vi "Query_Dust_Event_v2.vi"(8 "error in (no error)":errorcluster, 9 "Save Waveforms":bool) -> (0 "error out":errorcluster)   [LabVIEW 2013]
uses:
  Private/Constraints.ctl
  Private/Graph.ctl
  <vilib>/Utility/miscctls.llb/LVPointTypeDef.ctl
  <vilib>/Utility/error.llb/DialogType.ctl
  <userlib>/_OpenG.lib/array/array.llb/Remove Duplicates from 1D Array (String)__ogtk.vi
  <userlib>/_OpenG.lib/array/array.llb/Remove Duplicates from 1D Array (DBL)__ogtk.vi
  <vilib>/Utility/file.llb/Write To Spreadsheet File (string).vi
  Private/Global graph.vi
panel:
  out "Open plot windows":refnum<vi>[](array[refnum])
  out "Week":dbl
  out "Last Metadata Name":string
  out "Density":dbl
  out "Names":string[](array[string])
  in  "write metadata only":bool
  in  "Tab Control":T1(tab)
  in  "Limit to":dbl=10000.0
  in  "Limit plotted events":bool
  in  "Reset Scale to Default":bool
  in  "Experiment Group":string
  in  "Plot":bool
  in  "Select Names":bool
  in  "Save Metadata":bool
  in  "Show Names":bool
  out "Metadata Slide":u8(slide) scale=0.0..100.0
  in  "Save Image":bool
  in  "Plot Radius?":bool
  out "Constrained Distribution":T2
  in  "Experiment Name":string
  out "Waveforms Slide":u8(slide) scale=0.0..100.0
  in  "Reset Constraints to Default":bool
  in  "New Plot Window":bool
  out "Number of Matching Events:":i32
  out "Description for Experiment Name:":string caption="Experiment Description:"
  out "Percentage of triggers that fit constraints:":dbl format="%#_4g%"
  out "Total Number of triggers:":i64
  in  "Constraints":T3 {"Estimate Quality" scale=0.0..5.0; "Lower Mass Limit (kg)" min=0.0 step=1e-20; "Upper Mass Limit (kg)" min=0.0 step=1e-20}
  out "Dust Type":string
  in  "Radius (µm)":dbl=1.9999993051655787
  in  "Mass (kg)":dbl=2.6386e-13 min=1e-20 max=1e-10
  in  "Velocity (km/s)":dbl=1.0 min=0.1 max=200.0
  in  "Sensitivity:":dbl=12100000000000.0
  in  "Vnoise Estimate:":dbl=0.005
  in  "Pelletron Voltage (MV):":dbl=2.0
  out "Test":bool caption="Test Database in use:"
  out "Test 2":bool caption="Production Database in use:"
  in  "Exit":bool
  # "Query Dust Event 2.0"
  # "Cursor"
  # "events"
  # "Plot Settings:"
  # "Error Status:"
  # "ODBC Connection Status:"
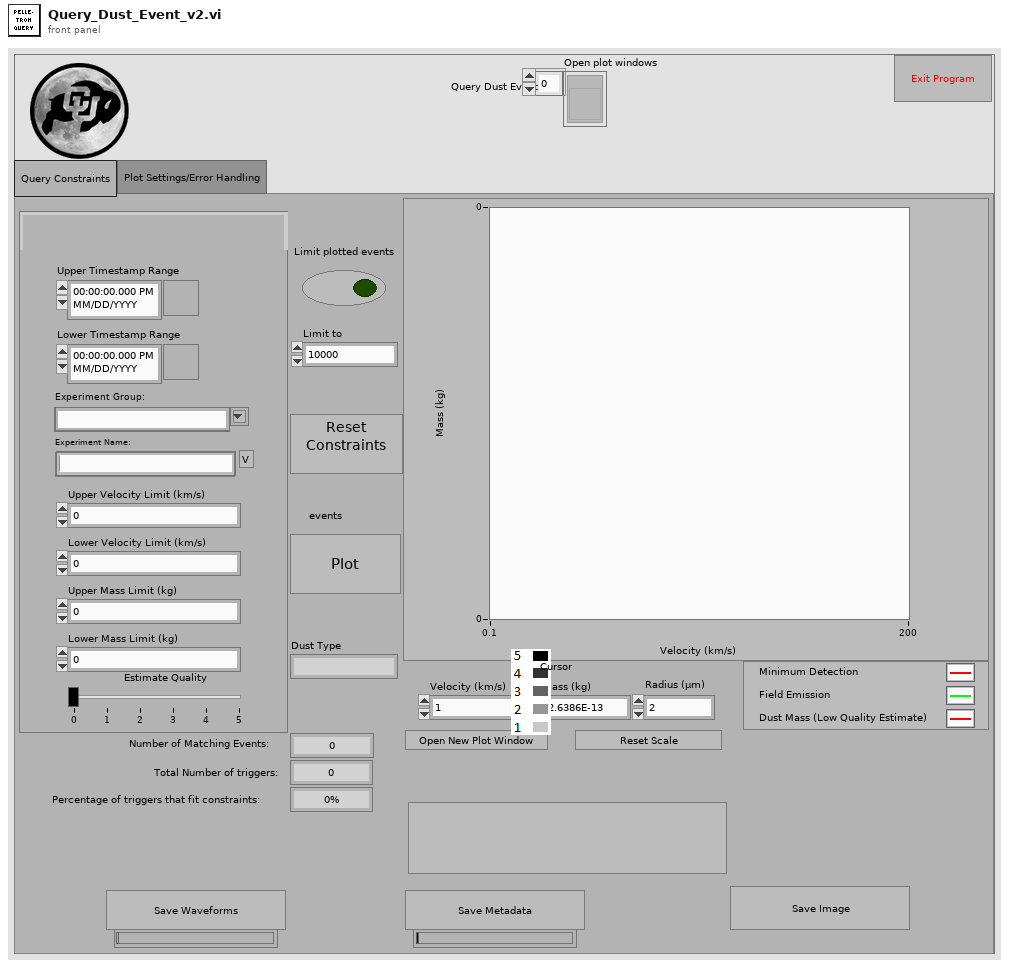
[diagram p1: front panel]
types:
  T1 = enum32{"Query Constraints", "Plot Settings/Error Handling"}
  T2 = typedef "Graph.ctl" = cluster{cluster{"Vnoise":dbl, "Vnoise":dbl}[]}[]
  T3 = typedef "Constraints.ctl" = cluster{"Upper Timestamp Range":timestamp, "Lower Timestamp Range":timestamp, "Experiment Group:":string, "Experiment Name:":i32[], "Upper Velocity Limit (km/s)":dbl, "Lower Velocity Limit (km/s)":dbl, "Upper Mass Limit (kg)":dbl, "Lower Mass Limit (kg)":dbl, "name array":string[], "Estimate Quality":cluster{dbl, dbl}}
  T4 = typedef "LVPointTypeDef.ctl" = cluster{"Horizontal":i16, "Vertical":i16}
  T5 = typedef "Query_Dust_Event.ctl" = cluster{"Dust Event ID":i64, "Integer Timestamp":i64, "Velocity":sgl, "Mass":sgl, "Charge":sgl, "Radius":sgl, "Passed_3rd_Detector":i8, "High Voltage":sgl, "+ High Voltage Supply":sgl, "- High Voltage Supply":sgl, "HV Control Difference":sgl, "Vacuum Pressure":sgl, "Radiation":sgl, "Column Current":sgl, "Lost Charge":sgl, "Chain Current":sgl, "Control High Voltage":sgl, "Current Group ID:":string, "Current Experiment Name:":string, "Current Experiment Description:":string, "Estimate Source":T6, "Estimate Quality":sgl, "File Location":T7, "Dust Type":string, "Dust Density":sgl}
  T6 = typedef "Estimate_source.ctl" = i8
  T7 = typedef "File_location.ctl" = i8
  T8 = enum8{"Enabled", "Disabled", "Disabled and Grayed Out"}
  T9 = enum16{"Left Button", "Center Button", "Right Button", "Window Close"}
  T10 = typedef "NI_Database_API.lvlib/Conn ObjectReference.ctl" = refnum<k1>
  T11 = typedef "DialogType.ctl" = u16
  T12 = typedef "Post_Signal.ctl" = cluster{"Integer Timestamp":i64, "Dust Event ID":i64, "Role ID":T13, "Data":sgl[], "Signal Length":i32, "dt":sgl, "Offset":dbl, "Hardware ID":T14}
  T13 = typedef "Role ID.ctl" = enum16{"First_Detector", "Second_Detector", "Third_Detector", "LeCroy_CH1", "LeCroy_CH2", "LeCroy_CH3", "LeCroy_CH4", "PSU"}
  T14 = typedef "Hardware ID.ctl" = enum16{"Unknown", "CSA 1", "CSA 2", "CSA 3", "CSA 4", "CSA 5", "CSA 6"}
  T15 = typedef "imagedata.ctl" = cluster{"image type":i32, "image depth":i32, "image":u8[], "mask":u8[], "colors":u32[], "Rectangle":cluster{"left":i16, "top":i16, "right":i16, "bottom":i16}}
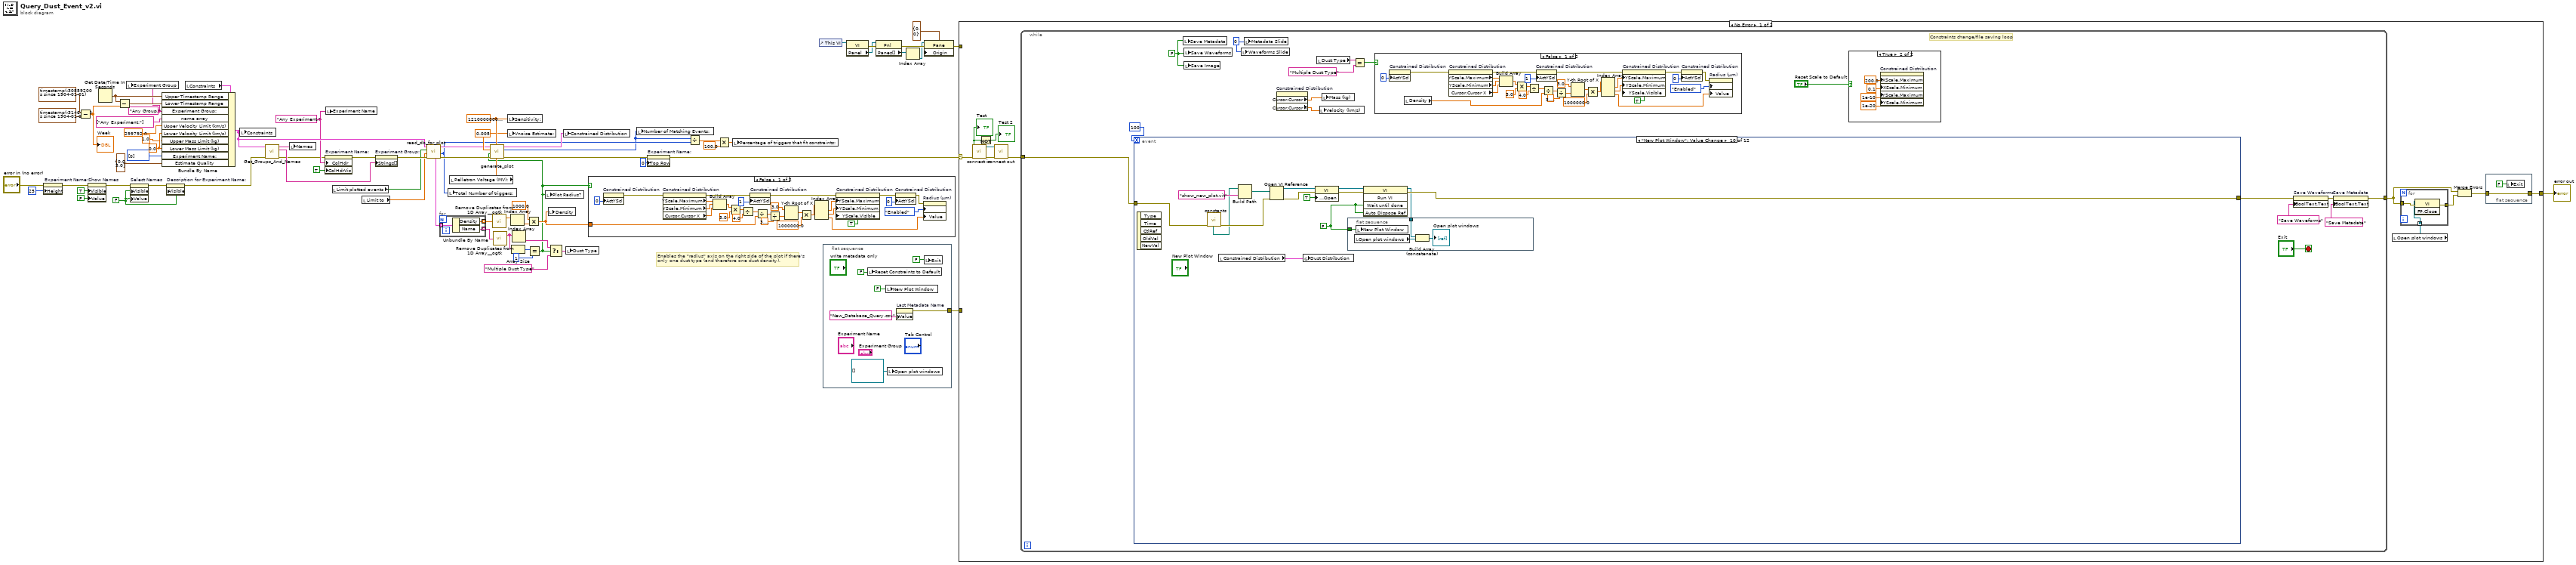
[diagram p0: block diagram]
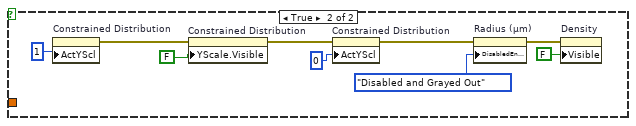
[diagram p2: hidden frame]
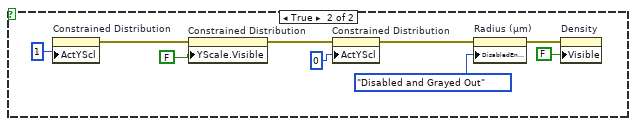
[diagram p3: hidden frame]
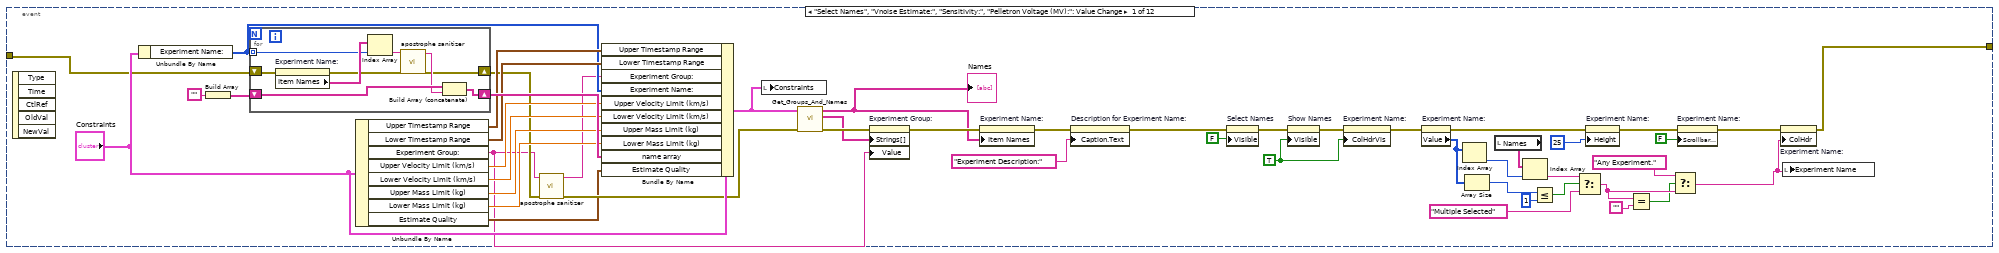
[diagram p5: hidden frame]
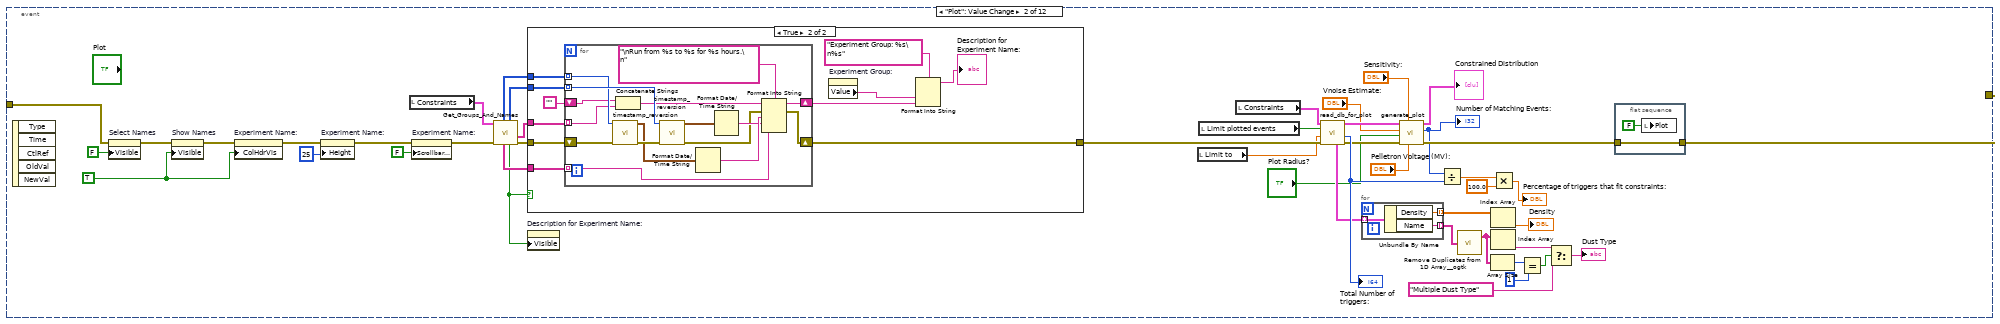
[diagram p6: hidden frame]
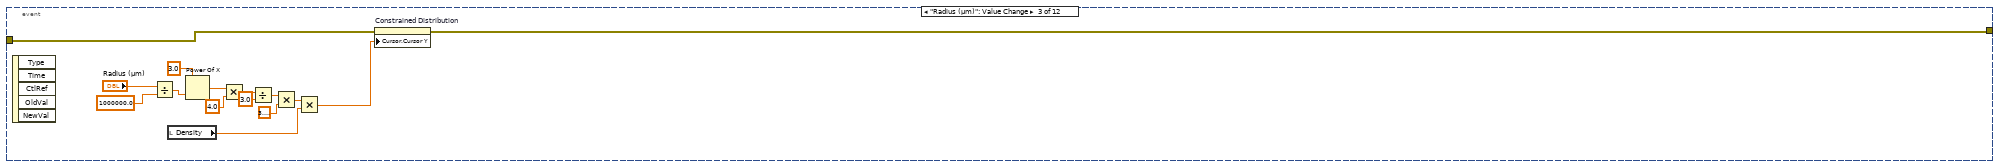
[diagram p8: hidden frame]
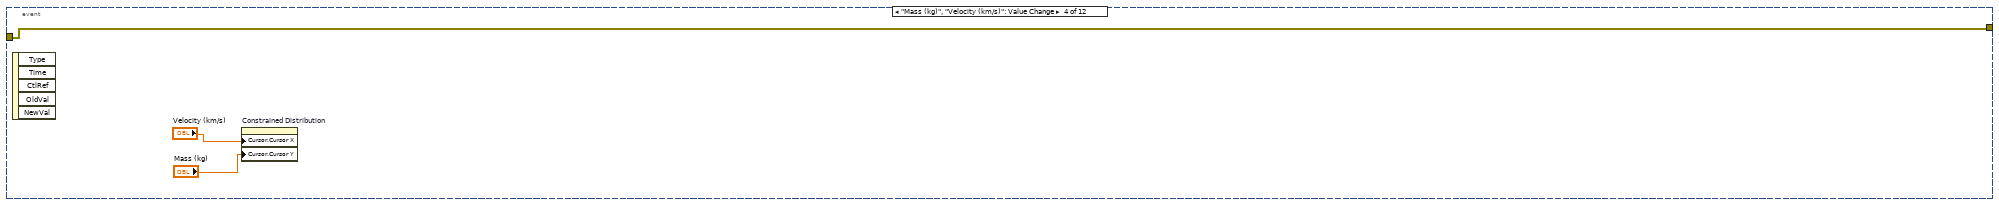
[diagram p9: hidden frame]
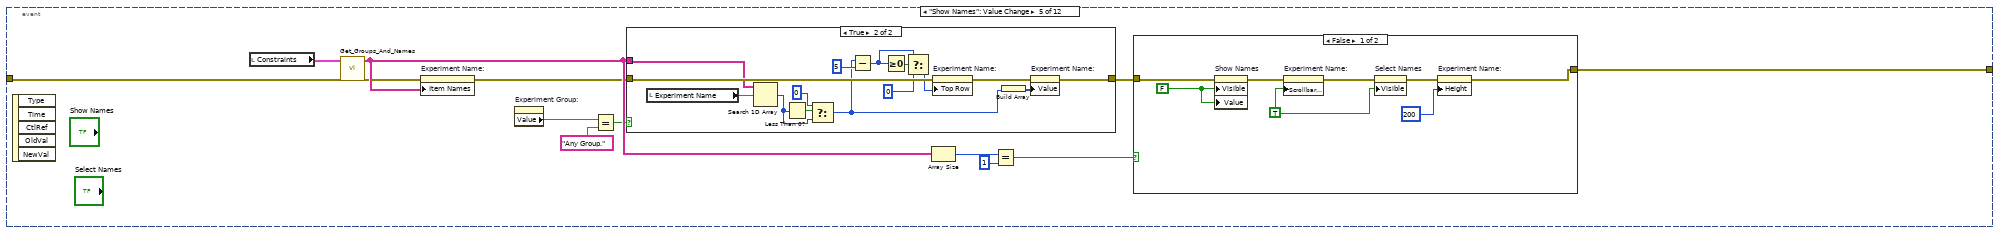
[diagram p10: hidden frame]
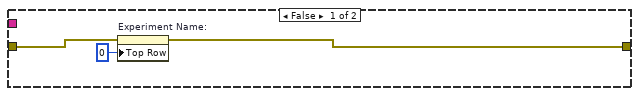
[diagram p11: hidden frame]
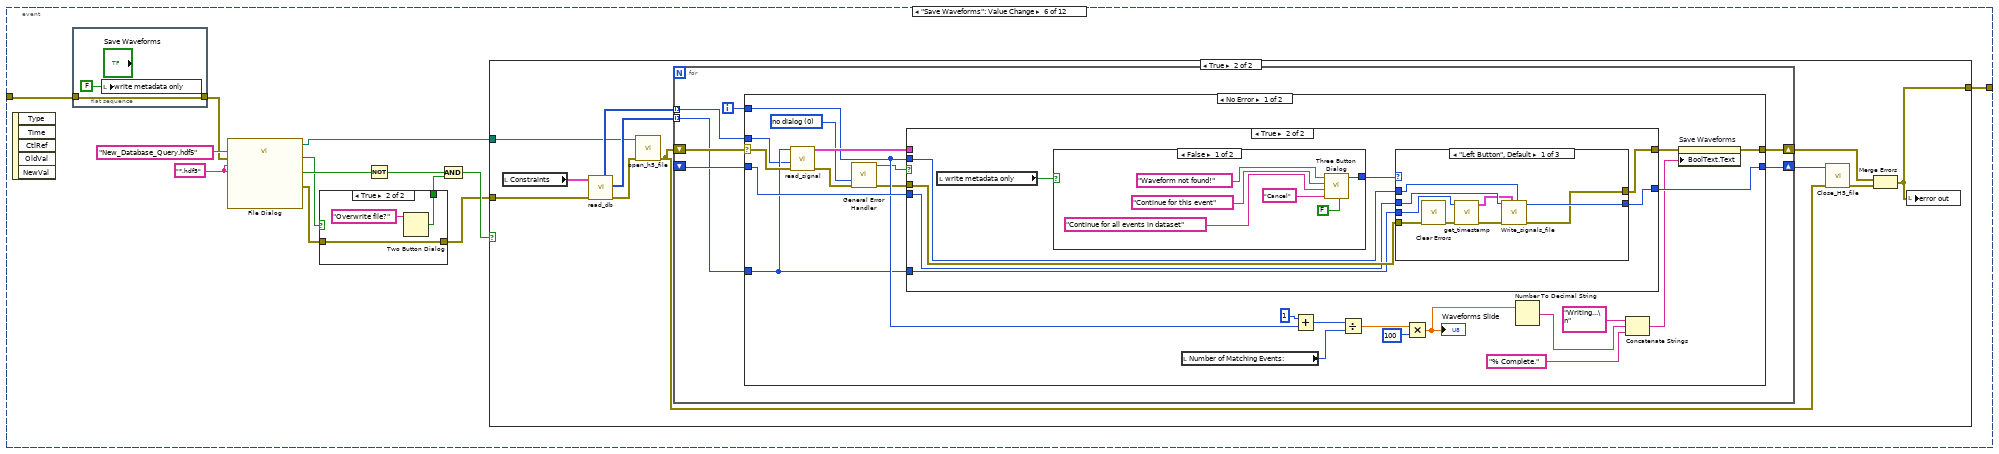
[diagram p13: hidden frame]
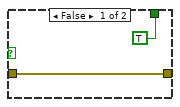
[diagram p14: hidden frame]
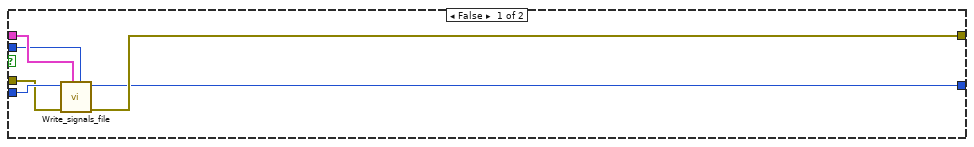
[diagram p16: hidden frame]
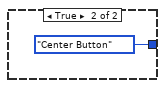
[diagram p17: hidden frame]
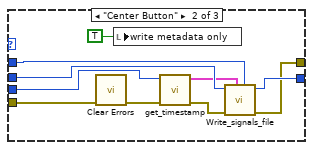
[diagram p18: hidden frame]
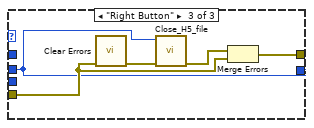
[diagram p19: hidden frame]
diagram:
  w12 = 0.0 ("Lower Mass Limit (kg)")
  w1 = "Any Group." ("element")
  w18 = FALSE ("Visible")
  w66 = 0.005 ("Vnoise")
  w67 = 12100000000000.0 ("Sens")
  w42 = "Any Experiment." ("element")
  # "Enables the \"radius\" axis on the right side of the plot if there's\nonly one dust type (and therefore one dust density)."
  n1 = property on="Experiment Name:" class="LstBox (strict)"(error in="error in (no error)", "Height"=25 ("x")) -> (error out=w15:errorcluster)  [unwired: 1 in, 1 out]
  n2 = Subtract(x=timestamp(-30859200 s since 1904-01-01) ("current time"), y=timestamp(-31464000 s since 1904-01-01) ("current time")) -> (x-y=w14:dbl)
  "Week" <- w14
  n3 = property on="Show Names" class="Bool (strict)"(error in=w15, "Visible"=TRUE, "Value"=FALSE ("Show Names")) -> (error out=w56:errorcluster)  [unwired: 1 in, 1 out]
  n4 = Get Date/Time In Seconds() -> (seconds since 1Jan1904=w59:timestamp)
  n5 = Subtract(x=w59, y=w14) -> (x-y=w58:timestamp)
  n6 = local write "Experiment Group"(w1) -> ()
  n7 = property on="Select Names" class="Bool (strict)"(error in=w56, "Visible"=w18, "Value"=w18) -> (error out=w55:errorcluster)  [unwired: 1 in, 1 out]
  n8 = property on="Description for Experiment Name:" class="Str"(error in=w55, "Visible"=w18) -> (error out=w33:errorcluster)  [unwired: 1 in, 1 out]
  n9 = local read "Constraints"() -> (w65:T3)
  n10 = Bundle By Name(cluster=w65, "Upper Timestamp Range"=w59, "Lower Timestamp Range"=w58, "Experiment Group:"=w1, "name array"=string[] ["Any Experiment."] ("Experiment Name:"), "Upper Velocity Limit (km/s)"=299792.0, "Lower Velocity Limit (km/s)"=w12, "Upper Mass Limit (kg)"=1.0 ("Lower Mass Limit (kg)"), "Lower Mass Limit (kg)"=w12, "Experiment Name:"=i32[] [0], "Estimate Quality"=cluster{dbl, dbl} {0.0, 5.0} ("Dust Quality")) -> (w46:T3)
  n11 = local write "Constraints"(w46) -> ()
  n12 = call "Get_Groups_And_Names.vi"("error in (no error)"=w33, "Constraints"=w46) -> ("error out"=w9:errorcluster, "Groups"=w70:string[], "Names"=w57:string[])  [unwired: 2 in, 5 out]
  n13 = local write "Names"(w57) -> ()
  n14 = property on="Experiment Name:" class="LstBox (strict)"(error in=w9, "ColHdr"=w42, "ColHdrVis"=TRUE ("Visible Items:Column Header Visible")) -> (error out=w53:errorcluster)  [unwired: 1 in, 1 out]
  n15 = local write "Experiment Name"(w42) -> ()
  n16 = local read "Limit plotted events"() -> (w8:bool)
  n17 = local read "Limit to"() -> (w7:dbl)
  n18 = property on="Experiment Group:" class="CmbBox"(error in=w53, "Strings[]"=w70) -> (error out=w69:errorcluster)  [unwired: 1 in, 1 out]
  n19 = call "read_db_for_plot.vi"("error in (no error)"=w69, "Limit no. of events"=w7, "Limited?"=w8, "Constraints"=w46) -> ("error out"=w68:errorcluster, "Total Number of events"=w48:i64, "Dust Array"=w62:T5[], "Dust Info"=w20:cluster{"Density":dbl, "Name":string}[])  [unwired: 3 in, 1 out]
  n20 = for {
    tunnel: w20 -> [w73] mode=indexing
    tunnel: [w72] -> w29 mode=indexing
    tunnel: [w71] -> w28 mode=indexing
    n21 = Unbundle By Name(w73) -> ("Density"=w72:dbl, "Name"=w71:string)
  }
  n22 = local write "Total Number of triggers:"(w48) -> ()
  n23 = local read "Pelletron Voltage (MV):"() -> (w63:dbl)
  n24 = call-poly <userlib>:"Remove Duplicates from 1D Array__ogtk.vi"("Input Array"=w29) -> ("Output Array"=w27:dbl[])  [unwired: 1 out]
  n25 = call-poly <userlib>:"Remove Duplicates from 1D Array__ogtk.vi"("Input Array"=w28) -> ("Output Array"=w26:string[])  [unwired: 1 out]
  n26 = local write "Sensitivity:"(w67) -> ()
  n27 = local write "Vnoise Estimate:"(w66) -> ()
  n28 = Index Array(array=w27) -> (element=w4:dbl)  [unwired: 1 in]
  n29 = Array Size(array=w26) -> (size(s)=w25:i32)
  n30 = Index Array(array=w26) -> (element=w22:string)  [unwired: 1 in]
  n31 = Multiply(x=1000.0 ("y"), y=w4) -> (x*y=w31:dbl)
  n32 = Equal?(x=w25, y=1) -> (x = y?=w6:bool)
  n33 = call "generate_plot.vi"("High Voltage"=w63, "Sens"=w67, "error in"=w68, "Plot Radius"=w6, "Vnoise"=w66, "Dust Array"=w62) -> ("error out"=w3:errorcluster, "Number of matching good events"=w47:i32, "Dust Distribution"=w64:T2)  [unwired: 3 in]
  n34 = local write "Plot Radius?"(w6) -> ()
  n35 = local write "Density"(w31) -> ()
  n36 = Select(t=w22, s=w6, f="Multiple Dust Type" ("t")) -> (s? t:f=w21:string)
  n37 = local write "Constrained Distribution"(w64) -> ()
  n38 = local write "Dust Type"(w21) -> ()
  n39 = case shown="False" w6 {
    tunnel: w31 -> [w80 _]
    frame False {
      n40 = property on="Constrained Distribution" class="XYGraph (strict)"("ActYScl"=0 ("Active Y Scale")) -> (error out=w94:errorcluster)  [unwired: 2 in, 1 out]
      n41 = property on="Constrained Distribution" class="XYGraph (strict)"(error in=w94) -> (error out=w92:errorcluster, "YScale.Maximum"=w87:dbl, "YScale.Minimum"=w86:dbl, "Cursor.Cursor X"=w74:dbl)  [unwired: 1 in, 1 out]
      n42 = Build Array(w87, w86, w74) -> (w85:dbl[])
      n43 = Multiply(x=w85, y=3.0) -> (x*y=w101:dbl[])
      n44 = Divide(x=w101, y=4.0) -> (x/y=w79:dbl[])
      n45 = property on="Constrained Distribution" class="XYGraph (strict)"(error in=w92, "ActYScl"=1 ("Active Y Scale")) -> (error out=w91:errorcluster)  [unwired: 1 in, 1 out]
      n46 = Divide(x=w79, y=w80) -> (x/y=w100:dbl[])
      n47 = Divide(x=w100, y=3.141592653589793) -> (x/y=w98:dbl[])
      n48 = Y-th Root of X(1:w98, 2:3.0 ("x")) -> (0:w97:dbl[])
      n49 = Multiply(x=w97, y=1000000.0) -> (x*y=w83:dbl[])
      n50 = Index Array(array=w83) -> (element #1=w84:dbl, element #2=w82:dbl, element #3=w75:dbl)  [unwired: 3 in]
      n51 = property on="Constrained Distribution" class="XYGraph (strict)"(error in=w91, "YScale.Maximum"=w84, "YScale.Minimum"=w82, "YScale.Visible"=TRUE ("Y Scale.Visible")) -> (error out=w76:errorcluster)  [unwired: 1 in, 1 out]
      n52 = property on="Constrained Distribution" class="XYGraph (strict)"(error in=w76, "ActYScl"=0 ("Active Y Scale")) -> (error out=w88:errorcluster)  [unwired: 1 in, 1 out]
      n53 = property on="Radius (µm)" class="DigNum (strict)"(error in=w88, "DisabledEnum"=T8."Enabled" ("Disabled"), "Value"=w75) -> ()  [unwired: 1 in, 2 out]
    }
    frame True {
      n54 = property on="Constrained Distribution" class="XYGraph (strict)"("ActYScl"=1 ("Active Y Scale")) -> (error out=w109:errorcluster)  [unwired: 2 in, 1 out]
      n55 = property on="Constrained Distribution" class="XYGraph (strict)"(error in=w109, "YScale.Visible"=FALSE ("Y Scale.Visible")) -> (error out=w107:errorcluster)  [unwired: 1 in, 1 out]
      n56 = property on="Constrained Distribution" class="XYGraph (strict)"(error in=w107, "ActYScl"=0 ("Active Y Scale")) -> (error out=w104:errorcluster)  [unwired: 1 in, 1 out]
      n57 = property on="Radius (µm)" class="DigNum (strict)"(error in=w104, "DisabledEnum"=T8."Disabled and Grayed Out" ("Disabled")) -> (error out=w103:errorcluster)  [unwired: 1 in, 1 out]
      n58 = property on="Density" class="DigNum (strict)"(error in=w103, "Visible"=FALSE) -> ()  [unwired: 1 in, 2 out]
    }
  }
  n59 = local write "Number of Matching Events:"(w47) -> ()
  n60 = property on="Experiment Name:" class="LstBox (strict)"(error in=w3, "Top Row"=0) -> (error out=w43:errorcluster)  [unwired: 1 in, 1 out]
  n61 = Divide(x=w47, y=w48) -> (x/y=w50:dbl)
  n62 = Multiply(x=w50, y=100.0) -> (x*y=w51:dbl)
  n63 = local write "Percentage of triggers that fit constraints:"(w51) -> ()
  n64 = control-ref of="This VI"() -> (w40:refnum<vi>)
  n65 = flat-sequence {
    tunnel: [w114] -> w30
    frame #0 {
      n66 = local write "Reset Constraints to Default"(FALSE) -> ()
      n67 = local write "New Plot Window"(FALSE ("write metadata only")) -> ()
      n68 = local write "Open plot windows"(refnum<vi>[] [] ("Open plot windows")) -> ()
      n69 = property on="Last Metadata Name" class="Str"("Value"="New_Database_Query.csv") -> (error out=w114:errorcluster)  [unwired: 2 in, 1 out]
      n70 = local write "Exit"(FALSE) -> ()
    }
  }
  n71 = property class="VI"(reference=w40) -> (error out=w39:errorcluster, "Panel"=w38:refnum<vi>)  [unwired: 1 in, 1 out]
  n72 = property class="Pnl"(reference=w38, error in=w39) -> (error out=w37:errorcluster, "Panes[]"=w36:refnum<vi>[])  [unwired: 1 out]
  n73 = Index Array(array=w36) -> (element=w35:refnum<vi>)  [unwired: 1 in]
  n74 = property class="Pane"(reference=w35, error in=w37, "Origin"=T4 {"Horizontal"=0, "Vertical"=0}) -> (error out=w2:errorcluster)  [unwired: 1 out]
  n75 = case shown="No Error" w43 {
    selector: w43 -> [w122 w645]
    tunnel: [w119 w645] -> w19
    tunnel: w30 -> [_ _]
    tunnel: w2 -> [_ _]
    frame No Error {
      n76 = call "connect in.vi"("error in (no error)"=w122) -> ("error out"=w126:errorcluster, "Database Connection"=w127:T10, "Test Server"=w121:bool)  [unwired: 6 in]
      "Test" <- w121
      n77 = Not(x=w121) -> (.not. x?=→"Test 2":bool)
      n78 = call "connect out.vi"("error in (no error)"=w126, "connection reference"=w127) -> ("error out"=w125:errorcluster)  [unwired: 9 in]
      n79 = while {
        tunnel: w125 -> [w147]
        tunnel: [w143] -> w124
        stop <- "Exit" stop-if-true
        w142 = u8 0 ("Slide")
        w134 = FALSE ("Save to File")
        # "Constraints change/file saving loop"
        n80 = event shown="[9] \"New Plot Window\": Value Change" {
          selector: _ -> [_ _ _ _ _ _ _ _ _ _ _ _]
          dyn-events: _ -> [_ _ _ _ _ _ _ _ _ _ _ _]
          timeout: 100 -> [_ _ _ _ _ _ _ _ _ _ _ _]
          tunnel: w147 -> [w221 w271 w329 w344 w352 w387 w507 w573 w584 w599 w624 w644]
          tunnel: [w208 w287 w330 w344 w359 w399 w508 w573 w582 w598 w623 w639] -> w146
          event "Select Names", "Vnoise Estimate:", "Sensitivity:", "Pelletron Voltage (MV):": Value Change {
            w217 = TRUE ("Visible")
            n81 = event-data() -> ()  [unwired: 1 in, 5 out]
            n82 = Unbundle By Name("Constraints") -> ("Experiment Name:"=w215:i32[])
            n83 = Build Array("") -> (w200:string[])
            n84 = for {
              tunnel: w215 -> [w248] mode=indexing
              shift-right: [w241] -> w239
              shift-left: w200 -> [w247]
              shift-right: [w242] -> w210
              shift-left: w221 -> [w246]
              n85 = property on="Experiment Name:" class="LstBox (strict)"(error in=w246) -> (error out=w243:errorcluster, "Item Names"=w249:string[])  [unwired: 1 in, 1 out]
              n86 = Index Array(array=w249, index=w248) -> (element=w245:string)
              n87 = call "apostrophe sanitizer.vi"("error in (no error)"=w243, "imput to db"=w245) -> ("error out"=w242:errorcluster, "fixed imput to db"=w244:string)  [unwired: 7 in, 1 out]
              n88 = Build Array (concatenate)(w247, w244) -> (w241:string[])
            }
            n89 = Unbundle By Name("Constraints") -> ("Upper Timestamp Range"=w238:timestamp, "Lower Timestamp Range"=w237:timestamp, "Experiment Group:"=w197:string, "Upper Velocity Limit (km/s)"=w236:dbl, "Lower Velocity Limit (km/s)"=w235:dbl, "Upper Mass Limit (kg)"=w234:dbl, "Lower Mass Limit (kg)"=w233:dbl, "Estimate Quality"=w203:cluster{dbl, dbl})
            n90 = call "apostrophe sanitizer.vi"("error in (no error)"=w210, "imput to db"=w197) -> ("error out"=w209:errorcluster, "fixed imput to db"=w211:string)  [unwired: 7 in, 1 out]
            n91 = Bundle By Name(cluster="Constraints", "Upper Timestamp Range"=w238, "Lower Timestamp Range"=w237, "Experiment Group:"=w211, "Experiment Name:"=w215, "Upper Velocity Limit (km/s)"=w236, "Lower Velocity Limit (km/s)"=w235, "Upper Mass Limit (kg)"=w234, "Lower Mass Limit (kg)"=w233, "name array"=w239, "Estimate Quality"=w203) -> (w198:T3)
            n92 = local write "Constraints"(w198) -> ()
            n93 = call "Get_Groups_And_Names.vi"("error in (no error)"=w209, "Constraints"=w198) -> ("error out"=w206:errorcluster, "Groups"=w205:string[], "Names"=w204:string[])  [unwired: 2 in, 5 out]
            "Names" <- w204
            n94 = property on="Experiment Group:" class="CmbBox"(error in=w206, "Strings[]"=w205, "Value"=w197) -> (error out=w219:errorcluster)  [unwired: 1 in, 1 out]
            n95 = property on="Experiment Name:" class="LstBox (strict)"(error in=w219, "Item Names"=w204) -> (error out=w218:errorcluster)  [unwired: 1 in, 1 out]
            n96 = property on="Description for Experiment Name:" class="Str"(error in=w218, "Caption.Text"="Experiment Description:" ("format string")) -> (error out=w207:errorcluster)  [unwired: 1 in, 1 out]
            n97 = property on="Select Names" class="Bool (strict)"(error in=w207, "Visible"=FALSE) -> (error out=w222:errorcluster)  [unwired: 1 in, 1 out]
            n98 = property on="Show Names" class="Bool (strict)"(error in=w222, "Visible"=w217) -> (error out=w202:errorcluster)  [unwired: 1 in, 1 out]
            n99 = property on="Experiment Name:" class="LstBox (strict)"(error in=w202, "ColHdrVis"=w217) -> (error out=w201:errorcluster)  [unwired: 1 in, 1 out]
            n100 = property on="Experiment Name:" class="LstBox (strict)"(error in=w201) -> (error out=w220:errorcluster, "Value"=w214:i32[])  [unwired: 1 in, 1 out]
            n101 = Index Array(array=w214) -> (element=w216:i32)  [unwired: 1 in]
            n102 = Array Size(array=w214) -> (size(s)=w228:i32)
            n103 = local read "Names"() -> (w227:string[])
            n104 = Index Array(array=w227, index=w216) -> (element=w212:string)
            n105 = Less Or Equal?(x=w228, y=1) -> (x <= y?=w229:bool)
            n106 = Select(t=w212, s=w229, f="Multiple Selected") -> (s? t:f=w193:string)
            n107 = property on="Experiment Name:" class="LstBox (strict)"(error in=w220, "Height"=u32 25 ("Size:Height")) -> (error out=w224:errorcluster)  [unwired: 1 in, 1 out]
            n108 = Equal?(x=w193, y="") -> (x = y?=w192:bool)
            n109 = Select(t="Any Experiment.", s=w192, f=w193) -> (s? t:f=w196:string)
            n110 = property on="Experiment Name:" class="LstBox (strict)"(error in=w224, "Scrollbar Visible"=FALSE ("Visible Items:Vertical Scrollbar Visible")) -> (error out=w226:errorcluster)  [unwired: 1 in, 1 out]
            n111 = property on="Experiment Name:" class="LstBox (strict)"(error in=w226, "ColHdr"=w196) -> (error out=w208:errorcluster)  [unwired: 1 in, 1 out]
            n112 = local write "Experiment Name"(w196) -> ()
          }
          event "Plot": Value Change {
            w293 = TRUE ("Visible")
            n113 = event-data() -> ()  [unwired: 1 in, 5 out]
            n114 = property on="Select Names" class="Bool (strict)"(error in=w271, "Visible"=FALSE) -> (error out=w290:errorcluster)  [unwired: 1 in, 1 out]
            n115 = property on="Show Names" class="Bool (strict)"(error in=w290, "Visible"=w293) -> (error out=w289:errorcluster)  [unwired: 1 in, 1 out]
            n116 = property on="Experiment Name:" class="LstBox (strict)"(error in=w289, "ColHdrVis"=w293) -> (error out=w269:errorcluster)  [unwired: 1 in, 1 out]
            n117 = property on="Experiment Name:" class="LstBox (strict)"(error in=w269, "Height"=u32 25 ("Size:Height")) -> (error out=w288:errorcluster)  [unwired: 1 in, 1 out]
            n118 = local read "Constraints"() -> (w270:T3)
            n119 = property on="Experiment Name:" class="LstBox (strict)"(error in=w288, "Scrollbar Visible"=FALSE ("Visible Items:Vertical Scrollbar Visible")) -> (error out=w257:errorcluster)  [unwired: 1 in, 1 out]
            n120 = call "Get_Groups_And_Names.vi"("error in (no error)"=w257, "Constraints"=w270) -> ("error out"=w256:errorcluster, "Description"=w253:string[], "Description Returned?"=w252:bool, "Run start integer timestamp"=w286:i64[], "Run Time (hrs)"=w284:string[], "Run stop integer timestamp"=w285:i64[])  [unwired: 2 in, 2 out]
            n121 = case shown="True" w252 {
              tunnel: w286 -> [_ w307]
              tunnel: w285 -> [_ w306]
              tunnel: w284 -> [_ w305]
              tunnel: [w296 w304] -> w275
              tunnel: w256 -> [w296 w298]
              tunnel: w253 -> [_ w297]
              frame False {
              }
              frame True {
                n122 = for {
                  tunnel: w297 -> [w310] mode=indexing
                  tunnel: w306 -> [w322] mode=indexing
                  tunnel: w307 -> [w323] mode=indexing
                  shift-right: [w312] -> w304
                  shift-left: w298 -> [w320]
                  shift-right: [w314] -> w302
                  shift-left: "" -> [w311]
                  tunnel: w305 -> [w309] mode=indexing
                  n123 = call "timestamp_reversion.vi"("error in (no error)"=w320, "Integer Timestamp"=w322) -> ("error out"=w321:errorcluster, "time stamp"=w318:timestamp)  [unwired: 7 in]
                  n124 = Concatenate Strings(w311, w310) -> (w308:string)
                  n125 = call "timestamp_reversion.vi"("error in (no error)"=w321, "Integer Timestamp"=w323) -> ("error out"=w313:errorcluster, "time stamp"=w319:timestamp)  [unwired: 7 in]
                  n126 = Format Date/Time String(seconds (now)=w318) -> (date/time string=w316:string)  [unwired: 2 in]
                  n127 = Format Date/Time String(seconds (now)=w319) -> (date/time string=w315:string)  [unwired: 2 in]
                  n128 = Format Into String(format string="\nRun from %s to %s for %s hours.\n", initial string=w308, error in=w313, w316, w315, w309) -> (resulting string=w314:string, error out=w312:errorcluster)
                }
                n129 = property on="Experiment Group:" class="CmbBox"() -> ("Value"=w301:string)  [unwired: 2 in, 2 out]
                n130 = Format Into String(format string="Experiment Group: %s\n%s", w301, w302) -> (resulting string=→"Description for Experiment Name:":string)  [unwired: 2 in, 1 out]
              }
            }
            n131 = property on="Description for Experiment Name:" class="Str"("Visible"=w252) -> ()  [unwired: 2 in, 2 out]
            n132 = local read "Limit to"() -> (w250:dbl)
            n133 = local read "Limit plotted events"() -> (w251:bool)
            n134 = local read "Constraints"() -> (w255:T3)
            n135 = call "read_db_for_plot.vi"("error in (no error)"=w275, "Limit no. of events"=w250, "Limited?"=w251, "Constraints"=w255) -> ("error out"=w276:errorcluster, "Total Number of events"=w277:i64, "Dust Array"=w278:T5[], "Dust Info"=w262:cluster{"Density":dbl, "Name":string}[])  [unwired: 3 in, 1 out]
            "Total Number of triggers:" <- w277
            n136 = for {
              tunnel: [w326] -> w259 mode=indexing
              tunnel: [w325] -> w268 mode=indexing
              tunnel: w262 -> [w324] mode=indexing
              n137 = Unbundle By Name(w324) -> ("Density"=w326:dbl, "Name"=w325:string)
            }
            n138 = call "generate_plot.vi"("High Voltage"="Pelletron Voltage (MV):", "Sens"="Sensitivity:", "error in"=w276, "Plot Radius"="Plot Radius?", "Vnoise"="Vnoise Estimate:", "Dust Array"=w278) -> ("error out"=w295:errorcluster, "Number of matching good events"=w279:i32, "Dust Distribution"=→"Constrained Distribution":T2)  [unwired: 3 in]
            "Number of Matching Events:" <- w279
            n139 = Divide(x=w279, y=w277) -> (x/y=w281:dbl)
            n140 = call-poly <userlib>:"Remove Duplicates from 1D Array__ogtk.vi"("Input Array"=w268) -> ("Output Array"=w260:string[])  [unwired: 1 out]
            n141 = Array Size(array=w260) -> (size(s)=w267:i32)
            n142 = Index Array(array=w259) -> (element=→"Density":dbl)  [unwired: 1 in]
            n143 = Index Array(array=w260) -> (element=w263:string)  [unwired: 1 in]
            n144 = Multiply(x=w281, y=100.0) -> (x*y=→"Percentage of triggers that fit constraints:":dbl)
            n145 = Equal?(x=w267, y=1) -> (x = y?=w264:bool)
            n146 = Select(t=w263, s=w264, f="Multiple Dust Type" ("t")) -> (s? t:f=→"Dust Type":string)
            n147 = flat-sequence {
              tunnel: [w327] -> w287
              tunnel: w295 -> [w327]
              frame #0 {
                n148 = local write "Plot"(FALSE ("Plot")) -> ()
              }
            }
          }
          event "Radius (µm)": Value Change {
            n149 = event-data() -> ()  [unwired: 1 in, 5 out]
            n150 = Divide(x="Radius (µm)", y=1000000.0) -> (x/y=w335:dbl)
            n151 = local read "Density"() -> (w332:dbl)
            n152 = Power Of X(1:w335, 2:3.0 ("y")) -> (0:w334:dbl)
            n153 = Multiply(x=w334, y=4.0) -> (x*y=w342:dbl)
            n154 = Divide(x=w342, y=3.0) -> (x/y=w340:dbl)
            n155 = Multiply(x=w340, y=3.141592653589793) -> (x*y=w333:dbl)
            n156 = Multiply(x=w333, y=w332) -> (x*y=w331:dbl)
            n157 = property on="Constrained Distribution" class="XYGraph (strict)"(error in=w329, "Cursor.Cursor Y"=w331) -> (error out=w330:errorcluster)  [unwired: 1 in, 1 out]
          }
          event "Mass (kg)", "Velocity (km/s)": Value Change {
            n158 = event-data() -> ()  [unwired: 1 in, 5 out]
            n159 = property on="Constrained Distribution" class="XYGraph (strict)"("Cursor.Cursor X"="Velocity (km/s)", "Cursor.Cursor Y"="Mass (kg)") -> ()  [unwired: 2 in, 2 out]
          }
          event "Show Names": Value Change {
            n160 = event-data() -> ()  [unwired: 1 in, 5 out]
            n161 = local read "Constraints"() -> (w355:T3)
            n162 = call "Get_Groups_And_Names.vi"("error in (no error)"=w352, "Constraints"=w355) -> ("error out"=w348:errorcluster, "Names"=w350:string[])  [unwired: 2 in, 6 out]
            n163 = property on="Experiment Name:" class="LstBox (strict)"(error in=w348, "Item Names"=w350) -> (error out=w347:errorcluster)  [unwired: 1 in, 1 out]
            n164 = property on="Experiment Group:" class="CmbBox"() -> ("Value"=w353:string)  [unwired: 2 in, 2 out]
            n165 = Equal?(x=w353, y="Any Group.") -> (x = y?=w349:bool)
            n166 = case shown="True" w349 {
              tunnel: w347 -> [w362 w377]
              tunnel: [w361 w374] -> w351
              tunnel: w350 -> [_ w370]
              frame False {
                n167 = property on="Experiment Name:" class="LstBox (strict)"(error in=w362, "Top Row"=0) -> (error out=w361:errorcluster)  [unwired: 1 in, 1 out]
              }
              frame True {
                n168 = local read "Experiment Name"() -> (w376:string)
                n169 = Search 1D Array(1D array=w370, element=w376) -> (index of element=w372:i32)  [unwired: 1 in]
                n170 = Less Than 0?(x=w372) -> (x < 0?=w373:bool)
                n171 = Select(t=0, s=w373, f=w372) -> (s? t:f=w366:i32)
                n172 = Subtract(x=w366, y=5) -> (x-y=w363:i32)
                n173 = Greater Or Equal To 0?(x=w363) -> (x >= 0?=w367:bool)
                n174 = Select(t=w363, s=w367, f=0) -> (s? t:f=w364:i32)
                n175 = property on="Experiment Name:" class="LstBox (strict)"(error in=w377, "Top Row"=w364) -> (error out=w375:errorcluster)  [unwired: 1 in, 1 out]
                n176 = Build Array(w366) -> (w369:i32[])
                n177 = property on="Experiment Name:" class="LstBox (strict)"(error in=w375, "Value"=w369) -> (error out=w374:errorcluster)  [unwired: 1 in, 1 out]
              }
            }
            n178 = Array Size(array=w350) -> (size(s)=w357:i32)
            n179 = Equal?(x=w357, y=1) -> (x = y?=w356:bool)
            n180 = case shown="False" w356 {
              tunnel: w351 -> [w385 w386]
              tunnel: [w383 w386] -> w359
              frame False {
                w378 = FALSE ("Visible")
                w382 = TRUE ("Visible Items:Vertical Scrollbar Visible")
                n181 = property on="Show Names" class="Bool (strict)"(error in=w385, "Visible"=w378, "Value"=w378) -> (error out=w381:errorcluster)  [unwired: 1 in, 1 out]
                n182 = property on="Experiment Name:" class="LstBox (strict)"(error in=w381, "Scrollbar Visible"=w382) -> (error out=w380:errorcluster)  [unwired: 1 in, 1 out]
                n183 = property on="Select Names" class="Bool (strict)"(error in=w380, "Visible"=w382) -> (error out=w384:errorcluster)  [unwired: 1 in, 1 out]
                n184 = property on="Experiment Name:" class="LstBox (strict)"(error in=w384, "Height"=200 ("x")) -> (error out=w383:errorcluster)  [unwired: 1 in, 1 out]
              }
              frame True {
              }
            }
          }
          event "Save Waveforms": Value Change {
            w395 = "*.hdf5"
            n185 = event-data() -> ()  [unwired: 1 in, 5 out]
            n186 = flat-sequence {
              tunnel: [w400] -> w388
              tunnel: w387 -> [w400]
              frame #0 {
                n187 = local write "write metadata only"(FALSE) -> ()
              }
            }
            n188 = call "File Dialog"("default name"="New_Database_Query.hdf5", "error in"=w388, "pattern (all files)"=w395, "pattern label"=w395) -> ("selected path"=w397:path, "exists"=w391:bool, "cancelled"=w398:bool, "error out"=w393:errorcluster)  [unwired: 8 in]
            n189 = case shown="True" w391 {
              tunnel: [w403 w406] -> w392
              tunnel: w393 -> [w403 w406]
              tunnel: [TRUE ("T button?") w405] -> w389
              frame False {
              }
              frame True {
                n190 = Two Button Dialog(message="Overwrite file?") -> (T button?=w405:bool)  [unwired: 2 in]
              }
            }
            n191 = Not(x=w398) -> (.not. x?=w390:bool)
            n192 = And(x=w390, y=w389) -> (x .and. y?=w394:bool)
            n193 = case shown="True" w394 {
              tunnel: [w407 w417] -> w399
              tunnel: w392 -> [w407 w411]
              tunnel: w397 -> [_ w410]
              frame False {
              }
              frame True {
                n194 = local read "Constraints"() -> (w408:T3)
                n195 = call "read_db.vi"("error in (no error)"=w411, "Constraints"=w408) -> ("error out"=w418:errorcluster, "Dust Event ID Array"=w413:i64[], "File Location Array"=w412:i64[])  [unwired: 5 in, 2 out]
                n196 = call "open_h5_file.vi"("error in (no error)"=w418, "path"=w410) -> ("error out"=w409:errorcluster)  [unwired: 8 in, 1 out]
                n197 = for {
                  tunnel: w413 -> [w421] mode=indexing
                  shift-right: [w425] -> w415
                  shift-left: w409 -> [w422]
                  shift-right: [w423] -> w414
                  shift-left: _ -> [w424]
                  tunnel: w412 -> [w419] mode=indexing
                  i -> [w420]
                  n198 = case shown="No Error" w422 {
                    selector: w422 -> [w437 w495]
                    tunnel: [w428 w495] -> w425
                    tunnel: w424 -> [w448 w494]
                    tunnel: [w446 w494] -> w423
                    tunnel: w421 -> [w435 _]
                    tunnel: w420 -> [w442 _]
                    tunnel: w419 -> [w426 _]
                    frame No Error {
                      w436 = T11 0 items=["no dialog", "OK message", "continue or stop message", "OK message + warnings", "continue/stop + warnings"] ("type of dialog (OK msg:1)")
                      n199 = call "read_signal.vi"("error in (no error)"=w437, "Location"=w426, "Dust Event ID"=w435) -> ("error out"=w439:errorcluster, "Signal Array"=w447:T12[])  [unwired: 7 in]
                      n200 = call <vilib>:"General Error Handler.vi"("type of dialog (OK msg:1)"=w436, "error in (no error)"=w439) -> ("error?"=w434:bool, "error out"=w438:errorcluster)  [unwired: 9 in, 3 out]
                      n201 = case shown="True" w434 {
                        tunnel: [w454 w456] -> w429
                        tunnel: w448 -> [w453 w459]
                        tunnel: w447 -> [w452 _]
                        tunnel: [w451 w458] -> w446
                        tunnel: w442 -> [w450 w460]
                        tunnel: w438 -> [w449 w462]
                        tunnel: w435 -> [_ w457]
                        frame False {
                          n202 = call "Write_signals_file.vi"("Index"=w450, "Signal Array"=w452, "error in (no error)"=w449, "ref"=w453) -> ("error out"=w454:errorcluster, "ref out"=w451:i32)  [unwired: 6 in]
                        }
                        frame True {
                          n203 = local read "write metadata only"() -> (w455:bool)
                          n204 = case shown="False" w455 {
                            tunnel: [w468 T9."Center Button" ("Which Button?")] -> w461
                            frame False {
                              n205 = call <vilib>:"Three Button Dialog.vi"("Allow user to close window? (TRUE)"=FALSE, "Right Button Text (\"Cancel\")"="Cancel" ("F button name (\"Cancel\")"), "Center Button Text (\"No\")"="Continue for all events in dataset" ("F button name (\"Cancel\")"), "Left Button Text (\"Yes\")"="Continue for this event" ("T button name (\"OK\")"), "message"="Waveform not found!") -> ("Which Button?"=w468:T9)  [unwired: 6 in]
                            }
                            frame True {
                            }
                          }
                          n206 = case shown="\"Left Button\", Default" w461 {
                            tunnel: w462 -> [w477 w487 w491]
                            tunnel: [w474 w484 w490] -> w456
                            tunnel: w459 -> [w475 w485 w489]
                            tunnel: w460 -> [w478 w488 _]
                            tunnel: [w476 w486 w489] -> w458
                            tunnel: w457 -> [w471 w481 _]
                            frame "Left Button", Default {
                              n207 = call <vilib>:"Clear Errors.vi"("error in (no error)"=w477) -> ("error out"=w472:errorcluster)  [unwired: 6 in]
                              n208 = call "get_timestamp.vi"("error in (no error)"=w472, "Index"=w471) -> ("error out"=w473:errorcluster, "Signal Array"=w470:T12[])  [unwired: 8 in]
                              n209 = call "Write_signals_file.vi"("Index"=w478, "Signal Array"=w470, "error in (no error)"=w473, "ref"=w475) -> ("error out"=w474:errorcluster, "ref out"=w476:i32)  [unwired: 6 in]
                            }
                            frame "Center Button" {
                              n210 = call <vilib>:"Clear Errors.vi"("error in (no error)"=w487) -> ("error out"=w482:errorcluster)  [unwired: 6 in]
                              n211 = local write "write metadata only"(TRUE) -> ()
                              n212 = call "get_timestamp.vi"("error in (no error)"=w482, "Index"=w481) -> ("error out"=w483:errorcluster, "Signal Array"=w480:T12[])  [unwired: 8 in]
                              n213 = call "Write_signals_file.vi"("Index"=w488, "Signal Array"=w480, "error in (no error)"=w483, "ref"=w485) -> ("error out"=w484:errorcluster, "ref out"=w486:i32)  [unwired: 6 in]
                            }
                            frame "Right Button" {
                              n214 = call <vilib>:"Clear Errors.vi"("error in (no error)"=w491) -> ("error out"=w493:errorcluster)  [unwired: 6 in]
                              n215 = call "Close_H5_file.vi"("error in (no error)"=w493, "ref"=w489) -> ("error out"=w492:errorcluster)  [unwired: 9 in]
                              n216 = Merge Errors(w492, w491) -> (w490:errorcluster)
                            }
                          }
                        }
                      }
                      n217 = local read "Number of Matching Events:"() -> (w445:i32)
                      n218 = Add(x=1, y=w442) -> (x+y=w441:i32)
                      n219 = Divide(x=w441, y=w445) -> (x/y=w444:dbl)
                      n220 = Multiply(x=w444, y=100) -> (x*y=w430:dbl)
                      "Waveforms Slide" <- w430
                      n221 = Number To Decimal String(number=w430) -> (decimal integer string=w433:string)  [unwired: 1 in]
                      n222 = Concatenate Strings("Writing...\n" ("string"), w433, "% Complete." ("string")) -> (w427:string)
                      n223 = property on="Save Waveforms" class="Bool (strict)"(error in=w429, "BoolText.Text"=w427) -> (error out=w428:errorcluster)  [unwired: 1 in, 1 out]
                    }
                    frame Error {
                    }
                  }
                }
                n224 = call "Close_H5_file.vi"("error in (no error)"=w409, "ref"=w414) -> ("error out"=w416:errorcluster)  [unwired: 9 in]
                n225 = Merge Errors(w415, w416) -> (w417:errorcluster)
                n226 = local write "error out"(w417) -> ()
              }
            }
          }
          event "Save Metadata": Value Change {
            w505 = "*.csv"
            n227 = event-data() -> ()  [unwired: 1 in, 5 out]
            n228 = local read "Last Metadata Name"() -> (w502:string)
            n229 = call "File Dialog"("default name"=w502, "error in"=w507, "pattern (all files)"=w505, "pattern label"=w505) -> ("selected path"=w504:path, "exists"=w501:bool, "cancelled"=w506:bool, "error out"=w500:errorcluster)  [unwired: 8 in]
            n230 = Strip Path(path=w504) -> (name=→"Last Metadata Name":string)  [unwired: 1 out]
            n231 = case shown="True" w501 {
              tunnel: [w510 w513] -> w499
              tunnel: w500 -> [w510 w513]
              tunnel: [TRUE ("T button?") w512] -> w496
              frame False {
              }
              frame True {
                n232 = Two Button Dialog(message="Overwrite file?") -> (T button?=w512:bool)  [unwired: 2 in]
              }
            }
            n233 = Not(x=w506) -> (.not. x?=w498:bool)
            n234 = And(x=w498, y=w496) -> (x .and. y?=w497:bool)
            n235 = case shown="True" w497 {
              tunnel: w504 -> [_ w527]
              tunnel: w499 -> [w514 w518]
              tunnel: [w514 w523] -> w508
              frame False {
              }
              frame True {
                n236 = property on="Save Metadata" class="Bool (strict)"(error in=w518, "BoolText.Text"="Querying Database\n(may take several mins)" ("Boolean Text.Text")) -> (error out=w517:errorcluster)  [unwired: 1 in, 1 out]
                n237 = local read "Constraints"() -> (w515:T3)
                n238 = call "read_db.vi"("error in (no error)"=w517, "Constraints"=w515) -> ("error out"=w524:errorcluster, "Dust Array"=w526:T5[])  [unwired: 5 in, 3 out]
                n239 = Array Size(array=w526) -> (size(s)=w525:i32)
                n240 = for {
                  tunnel: w526 -> [w572] mode=indexing
                  tunnel: w525 -> [w558]
                  shift-right: [w557] -> w523
                  shift-left: w524 -> [w548]
                  tunnel: [w544] -> w520 mode=indexing
                  i -> [w529]
                  w535 = "\" %s \"" ("format string")
                  w533 = "%Y%m%d%H%M%S%9u" ("time format string (%c)")
                  n241 = Unbundle By Name(w572) -> ("Dust Event ID"=w556:i64, "Integer Timestamp"=w549:i64, "Velocity"=w555:sgl, "Mass"=w554:sgl, "Charge"=w550:sgl, "Radius"=w553:sgl, "High Voltage"=w552:sgl, "Current Group ID:"=w539:string, "Current Experiment Name:"=w541:string, "Current Experiment Description:"=w543:string, "Estimate Quality"=w551:sgl, "Dust Type"=w537:string)
                  n242 = Increment(x=w529) -> (x+1=w528:i32)
                  n243 = Divide(x=w528, y=w558) -> (x/y=w559:dbl)
                  n244 = Multiply(x=w559, y=100) -> (x*y=w546:dbl)
                  "Metadata Slide" <- w546
                  n245 = Number To Decimal String(number=w546) -> (decimal integer string=w561:string)  [unwired: 1 in]
                  n246 = Concatenate Strings("Writing...\n" ("string"), w561, "% Complete." ("string")) -> (w564:string)
                  n247 = call "timestamp_reversion.vi"("error in (no error)"=w548, "Integer Timestamp"=w549) -> ("error out"=w547:errorcluster, "time stamp"=w532:timestamp)  [unwired: 7 in]
                  n248 = Format Into String(format string=w535, w539) -> (resulting string=w538:string)  [unwired: 2 in, 1 out]
                  n249 = Format Into String(format string=w535, w541) -> (resulting string=w540:string)  [unwired: 2 in, 1 out]
                  n250 = Format Into String(format string=w535, w543) -> (resulting string=w542:string)  [unwired: 2 in, 1 out]
                  n251 = Format Into String(format string=w535, w537) -> (resulting string=w536:string)  [unwired: 2 in, 1 out]
                  n252 = Format Date/Time String(time format string (%c)=w533, seconds (now)=w532) -> (date/time string=w545:string)  [unwired: 1 in]
                  n253 = Number To Decimal String(number=w556) -> (decimal integer string=w534:string)  [unwired: 1 in]
                  n254 = Number To Decimal String(number=w549) -> (decimal integer string=w571:string)  [unwired: 1 in]
                  n255 = Number To Exponential String(number=w555) -> (E-format string=w570:string)  [unwired: 3 in]
                  n256 = Number To Exponential String(number=w554) -> (E-format string=w569:string)  [unwired: 3 in]
                  n257 = Number To Exponential String(number=w550) -> (E-format string=w568:string)  [unwired: 3 in]
                  n258 = Number To Exponential String(number=w553) -> (E-format string=w567:string)  [unwired: 3 in]
                  n259 = Number To Exponential String(number=w552) -> (E-format string=w566:string)  [unwired: 3 in]
                  n260 = Number To Decimal String(number=w551) -> (decimal integer string=w565:string)  [unwired: 1 in]
                  n261 = Format Date/Time String(time format string (%c)=w533, seconds (now)=w532, UTC format=TRUE) -> (date/time string=w530:string)
                  n262 = property on="Save Metadata" class="Bool (strict)"(error in=w547, "BoolText.Text"=w564) -> (error out=w557:errorcluster)  [unwired: 1 in, 1 out]
                  n263 = Build Array(w534, w530, w545, w571, w570, w569, w568, w567, w566, w538, w540, w542, w565, w536) -> (w544:string[])
                }
                n264 = Build Array (concatenate)(string[] ["Dust Event ID", "UTC Timestamp", "Local Timestamp", "Integer Timestamp (ms)", "Velocity (m/s)", "Mass (kg)", "Charge (C)", "Radius (m) ", "High Voltage (MV)", "Current Group ID", "Current Experiment Name", "Current Experiment Description", "Estimate Quality", "Dust Type", "Dust Type", "Dust Type"], w520) -> (w519:string[][])
                n265 = call-poly <vilib>:"Write To Spreadsheet File.vi"("delimiter (\\t)"="," ("delimiter (\\t)"), "2D data"=w519, "file path (dialog if empty)"=w527) -> ()  [unwired: 5 in, 1 out]
              }
            }
          }
          event Timeout {
            n266 = event-data() -> ()  [unwired: 1 in, 2 out]
          }
          event "Save Image": Value Change {
            w578 = "*.png"
            n267 = event-data() -> ()  [unwired: 1 in, 5 out]
            n268 = invoke on="Constrained Distribution" class="XYGraph (strict)" method="Get Image"(error in=w584) -> (error out=w579:errorcluster, "image data"=w583:T15)  [unwired: 5 in, 4 out]
            n269 = call "File Dialog"("default name"="Distribution.png", "error in"=w579, "pattern (all files)"=w578, "pattern label"=w578) -> ("selected path"=w581:path, "exists"=w575:bool, "error out"=w576:errorcluster)  [unwired: 8 in, 1 out]
            n270 = case shown="True" w575 {
              tunnel: [w591 w594] -> w577
              tunnel: w576 -> [w591 w594]
              tunnel: [TRUE ("T button?") w593] -> w574
              frame False {
              }
              frame True {
                n271 = Two Button Dialog(message="Overwrite file?") -> (T button?=w593:bool)  [unwired: 2 in]
              }
            }
            n272 = case shown="True" w574 {
              tunnel: w583 -> [_ w589]
              tunnel: [w585 w588] -> w582
              tunnel: w581 -> [_ w587]
              tunnel: w577 -> [w585 w586]
              frame False {
              }
              frame True {
                n273 = call <vilib>:"Write PNG File.vi"("error in (no error)"=w586, "image data"=w589, "path to PNG file"=w587) -> ("error out"=w588:errorcluster)  [unwired: 7 in, 1 out]
              }
            }
          }
          event "New Plot Window": Value Change {
            w597 = FALSE ("Wait Until Done")
            n274 = event-data() -> ()  [unwired: 1 in, 5 out]
            n275 = call "constants.vi"("error in (no error)"=w599) -> ("error out"=w607:errorcluster, "Private Folder file path"=w604:path)  [unwired: 4 in, 5 out]
            n276 = local read "Constrained Distribution"() -> (w596:T2)
            n277 = Build Path(base path=w604, name or relative path="show_new_plot.vit") -> (appended path=w605:path)
            n278 = Open VI Reference(vi path=w605, error in (no error)=w607) -> (vi reference=w603:refnum<vi>, error out=w608:errorcluster)  [unwired: 4 in]
            n279 = global write "Global graph.vi" "Dust Distribution"(w596) -> ()
            n280 = property class="VI"(reference=w603, error in=w608, "Front Panel.Open"=TRUE ("Front Panel Window:Open")) -> (reference out=w600:refnum<vi>, error out=w601:errorcluster)
            n281 = flat-sequence {
              tunnel: w597 -> [w610]
              tunnel: w595 -> [w612]
              frame #0 {
                n282 = local read "Open plot windows"() -> (w609:refnum<vi>[])
                n283 = local write "New Plot Window"(w610) -> ()
                n284 = Build Array (concatenate)(w612, w609) -> (→"Open plot windows":refnum<vi>[])
              }
            }
            n285 = invoke class="VI" method="Run VI"(reference=w600, error in=w601, "Wait until done"=w597, "Auto Dispose Ref"=w597) -> (reference out=w595:refnum<vi>, error out=w598:errorcluster)  [unwired: 1 in, 3 out]
          }
          event "Reset Constraints to Default": Value Change {
            w619 = "Any Group." ("Experiment Group")
            w628 = FALSE ("Visible")
            w617 = "Any Experiment." ("element")
            n286 = event-data() -> ()  [unwired: 1 in, 6 out]
            n287 = local read "Constraints"() -> (w621:T3)
            n288 = Unbundle By Name(w621) -> ("Upper Velocity Limit (km/s)"=w636:dbl, "Lower Velocity Limit (km/s)"=w635:dbl, "Upper Mass Limit (kg)"=w634:dbl, "Lower Mass Limit (kg)"=w633:dbl, "Estimate Quality"=w620:cluster{dbl, dbl})
            n289 = local read "Week"() -> (w613:dbl)
            n290 = Get Date/Time In Seconds() -> (seconds since 1Jan1904=w627:timestamp)
            n291 = property on="Experiment Name:" class="LstBox (strict)"("ColHdr"=w617, "Height"=u32 25 ("Size:Height")) -> ()  [unwired: 2 in, 2 out]
            n292 = local write "Experiment Name"(w617) -> ()
            n293 = Build Array(w617) -> (w616:string[])
            n294 = local write "Experiment Group"(w619) -> ()
            n295 = Subtract(x=w627, y=w613) -> (x-y=w626:timestamp)
            n296 = Bundle By Name(cluster=w621, "Upper Timestamp Range"=w627, "Lower Timestamp Range"=w626, "Experiment Group:"=w619, "Experiment Name:"=i32[] [], "Upper Velocity Limit (km/s)"=w636, "Lower Velocity Limit (km/s)"=w635, "Upper Mass Limit (kg)"=w634, "Lower Mass Limit (kg)"=w633, "name array"=w616, "Estimate Quality"=w620) -> (w614:T3)
            n297 = property on="Select Names" class="Bool (strict)"("Visible"=w628, "Value"=w628) -> ()  [unwired: 2 in, 2 out]
            n298 = property on="Show Names" class="Bool (strict)"("Visible"=TRUE, "Value"=w628) -> ()  [unwired: 2 in, 2 out]
            n299 = local write "Constraints"(w614) -> ()
            n300 = call "Get_Groups_And_Names.vi"("error in (no error)"=w624, "Constraints"=w614) -> ("error out"=w631:errorcluster, "Groups"=w632:string[], "Names"=w625:string[])  [unwired: 2 in, 5 out]
            n301 = property on="Experiment Group:" class="CmbBox"(error in=w631, "Strings[]"=w632) -> (error out=w630:errorcluster)  [unwired: 1 in, 1 out]
            n302 = property on="name array" class="Arr (strict)"(error in=w630, "Value"=w625) -> (error out=w622:errorcluster)  [unwired: 1 in, 1 out]
            n303 = flat-sequence {
              tunnel: [w637] -> w623
              tunnel: w622 -> [w637]
              frame #0 {
                n304 = property on="Reset Constraints to Default" class="Bool (strict)"("Value"=FALSE ("Reset Constraints to Default")) -> ()  [unwired: 2 in, 2 out]
              }
            }
          }
          event "Limit plotted events": Value Change {
            n305 = event-data() -> ()  [unwired: 1 in, 6 out]
            n306 = Select(t=T8."Enabled" ("Disabled"), s="Limit plotted events", f=T8."Disabled and Grayed Out" ("Disabled")) -> (s? t:f=w640:T8)
            n307 = property on="Limit to" class="DigNum (strict)"(error in=w644, "DisabledEnum"=w640) -> (error out=w639:errorcluster)  [unwired: 1 in, 1 out]
          }
        }
        n308 = local write "Save Metadata"(w134) -> ()
        n309 = local write "Save Waveforms"(w134) -> ()
        n310 = local write "Save Image"(w134) -> ()
        n311 = local write "Waveforms Slide"(w142) -> ()
        n312 = local write "Metadata Slide"(w142) -> ()
        n313 = property on="Constrained Distribution" class="XYGraph (strict)"() -> ("Cursor.Cursor Y"=w138:dbl, "Cursor.Cursor X"=w139:dbl)  [unwired: 2 in, 2 out]
        n314 = local read "Dust Type"() -> (w141:string)
        n315 = local write "Velocity (km/s)"(w139) -> ()
        n316 = local write "Mass (kg)"(w138) -> ()
        n317 = Equal?(x=w141, y="Multiple Dust Type" ("t")) -> (x = y?=w135:bool)
        n318 = case shown="False" w135 {
          frame False {
            n319 = property on="Constrained Distribution" class="XYGraph (strict)"("ActYScl"=0 ("Active Y Scale")) -> (error out=w170:errorcluster)  [unwired: 2 in, 1 out]
            n320 = local read "Density"() -> (w150:dbl)
            n321 = property on="Constrained Distribution" class="XYGraph (strict)"(error in=w170) -> (error out=w168:errorcluster, "YScale.Maximum"=w163:dbl, "YScale.Minimum"=w162:dbl, "Cursor.Cursor X"=w151:dbl)  [unwired: 1 in, 1 out]
            n322 = Build Array(w163, w162, w151) -> (w161:dbl[])
            n323 = Multiply(x=w161, y=3.0) -> (x*y=w177:dbl[])
            n324 = Divide(x=w177, y=4.0) -> (x/y=w156:dbl[])
            n325 = property on="Constrained Distribution" class="XYGraph (strict)"(error in=w168, "ActYScl"=1 ("Active Y Scale")) -> (error out=w167:errorcluster)  [unwired: 1 in, 1 out]
            n326 = Divide(x=w156, y=w150) -> (x/y=w176:dbl[])
            n327 = Divide(x=w176, y=3.141592653589793) -> (x/y=w174:dbl[])
            n328 = Y-th Root of X(1:w174, 2:3.0 ("x")) -> (0:w173:dbl[])
            n329 = Multiply(x=w173, y=1000000.0) -> (x*y=w159:dbl[])
            n330 = Index Array(array=w159) -> (element #1=w160:dbl, element #2=w158:dbl, element #3=w152:dbl)  [unwired: 3 in]
            n331 = property on="Constrained Distribution" class="XYGraph (strict)"(error in=w167, "YScale.Maximum"=w160, "YScale.Minimum"=w158, "YScale.Visible"=TRUE ("Y Scale.Visible")) -> (error out=w153:errorcluster)  [unwired: 1 in, 1 out]
            n332 = property on="Constrained Distribution" class="XYGraph (strict)"(error in=w153, "ActYScl"=0 ("Active Y Scale")) -> (error out=w164:errorcluster)  [unwired: 1 in, 1 out]
            n333 = property on="Radius (µm)" class="DigNum (strict)"(error in=w164, "DisabledEnum"=T8."Enabled" ("Disabled"), "Value"=w152) -> ()  [unwired: 1 in, 2 out]
          }
          frame True {
            n334 = property on="Constrained Distribution" class="XYGraph (strict)"("ActYScl"=1 ("Active Y Scale")) -> (error out=w185:errorcluster)  [unwired: 2 in, 1 out]
            n335 = property on="Constrained Distribution" class="XYGraph (strict)"(error in=w185, "YScale.Visible"=FALSE ("Y Scale.Visible")) -> (error out=w183:errorcluster)  [unwired: 1 in, 1 out]
            n336 = property on="Constrained Distribution" class="XYGraph (strict)"(error in=w183, "ActYScl"=0 ("Active Y Scale")) -> (error out=w180:errorcluster)  [unwired: 1 in, 1 out]
            n337 = property on="Radius (µm)" class="DigNum (strict)"(error in=w180, "DisabledEnum"=T8."Disabled and Grayed Out" ("Disabled")) -> (error out=w179:errorcluster)  [unwired: 1 in, 1 out]
            n338 = property on="Density" class="DigNum (strict)"(error in=w179, "Visible"=FALSE) -> ()  [unwired: 1 in, 2 out]
          }
        }
        n339 = case shown="True" "Reset Scale to Default" {
          frame False {
          }
          frame True {
            n340 = property on="Constrained Distribution" class="XYGraph (strict)"("XScale.Maximum"=200.0 ("X Scale.Range:Maximum"), "XScale.Minimum"=0.1 ("X Scale.Range:Minimum"), "YScale.Maximum"=1e-10 ("Y Scale.Range:Maximum"), "YScale.Minimum"=1e-20 ("Y Scale.Range:Minimum")) -> ()  [unwired: 2 in, 2 out]
          }
        }
        n341 = property on="Save Waveforms" class="Bool (strict)"(error in=w146, "BoolText.Text"="Save Waveforms" ("f")) -> (error out=w144:errorcluster)  [unwired: 1 in, 1 out]
        n342 = property on="Save Metadata" class="Bool (strict)"(error in=w144, "BoolText.Text"="Save Metadata" ("Boolean Text.Text")) -> (error out=w143:errorcluster)  [unwired: 1 in, 1 out]
      }
      n343 = local read "Open plot windows"() -> (w118:refnum<vi>[])
      n344 = for {
        tunnel: w124 -> [w133]
        tunnel: [w132] -> w123
        tunnel: w118 -> [w131] mode=indexing
        n345 = invoke class="VI" method="FP.Close"(reference=w131, error in=w133) -> (error out=w132:errorcluster)  [unwired: 1 in, 2 out]
      }
      n346 = Merge Errors(w124, w123) -> (w120:errorcluster)
      n347 = flat-sequence {
        tunnel: w120 -> [w130]
        tunnel: [w130] -> w119
        frame #0 {
          n348 = local write "Exit"(FALSE ("Exit")) -> ()
        }
      }
    }
    frame Error {
    }
  }
  "error out" <- w19
